vi "copyFileByFileDate.vi"() -> ()   [LabVIEW 2012]
panel:
  out "folder names":string[](array[string])
  out "filenames":string[](array[string])
  out "?":string
  out "stripped path":path
  in  "Run":bool
  out "Source":path
  out "Destination":path
  in  "path":path=path "G:/DCIM"
  in  "Target Disk":string="d:"
  in  "JPG ?":string="JPG"
  out "folder names 3":string[](array[string])
  out "filenames 3":string[](array[string])
  out "path out 3":path
  out "array":string[][](array[string])
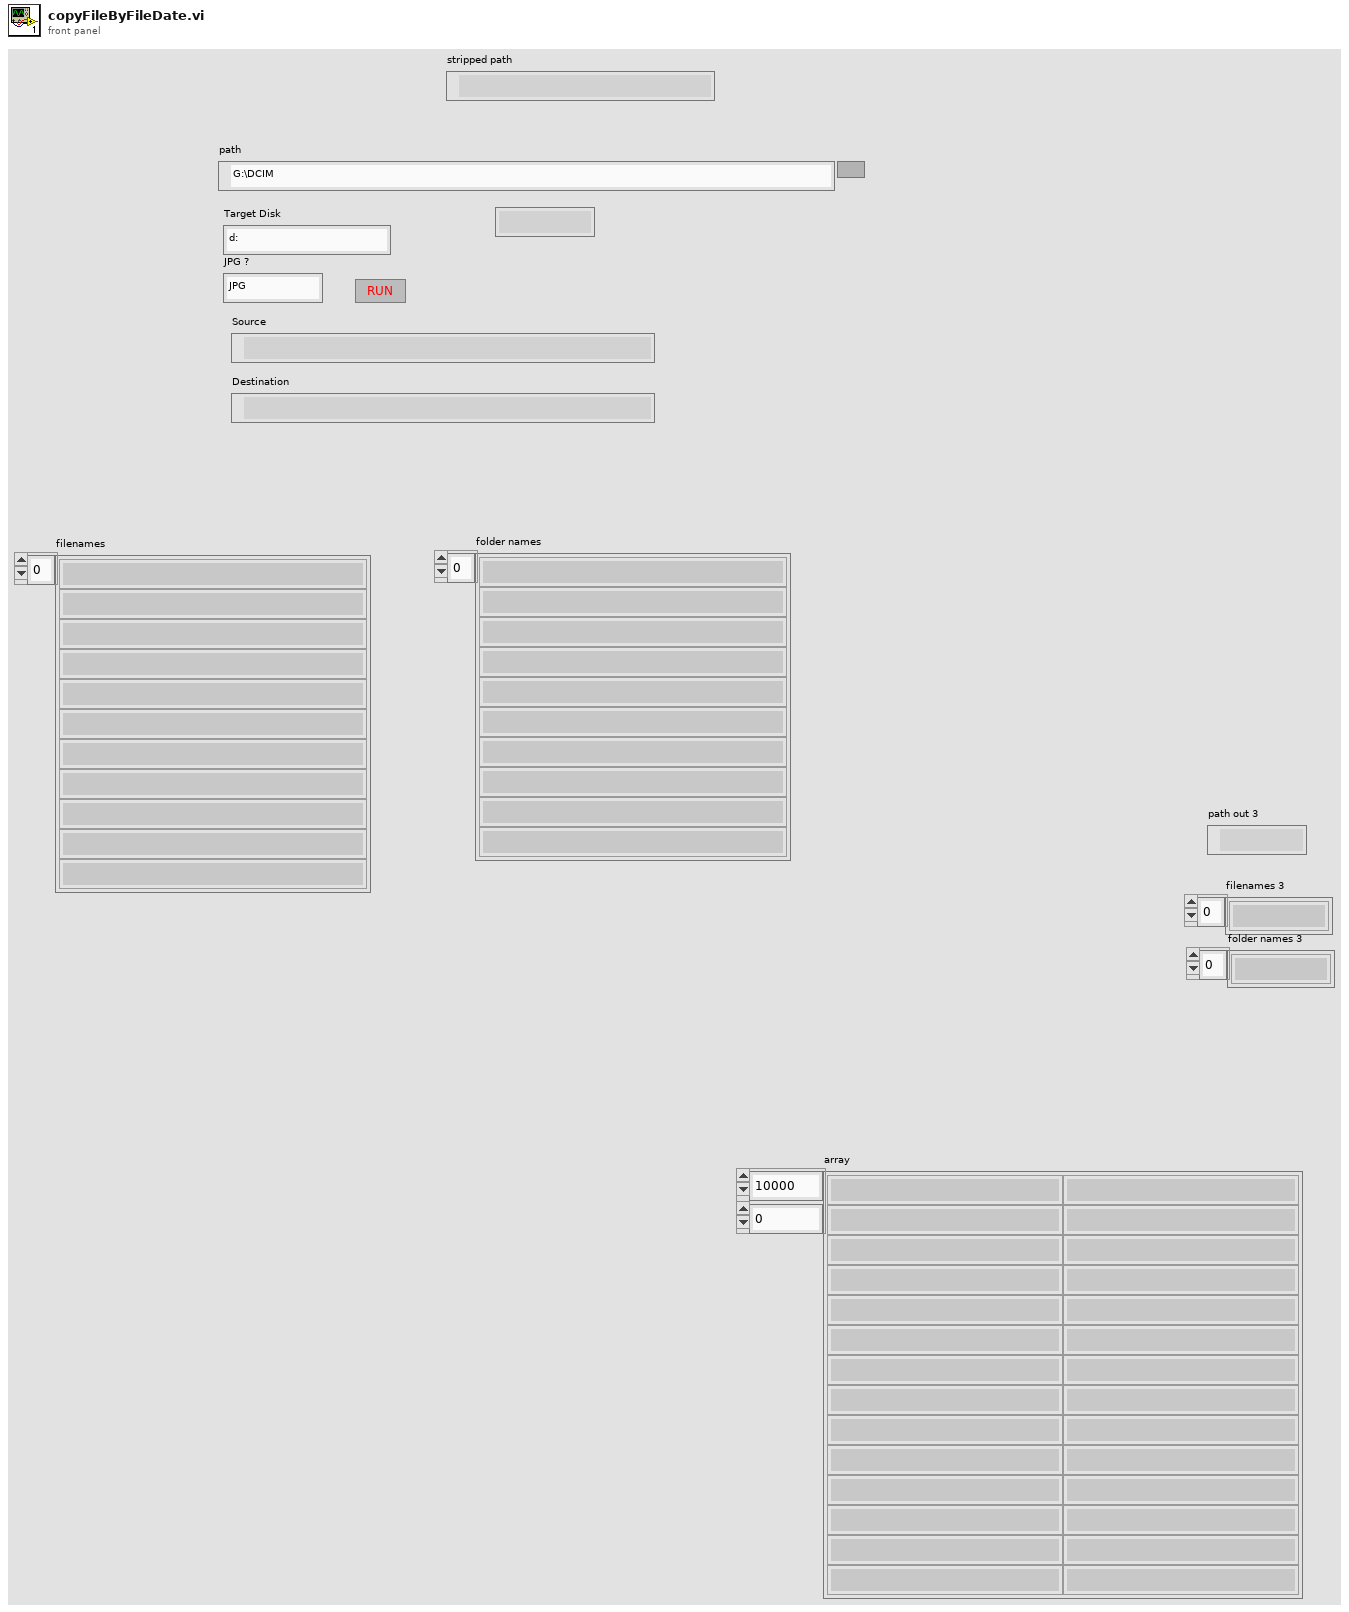
[diagram p1: front panel]
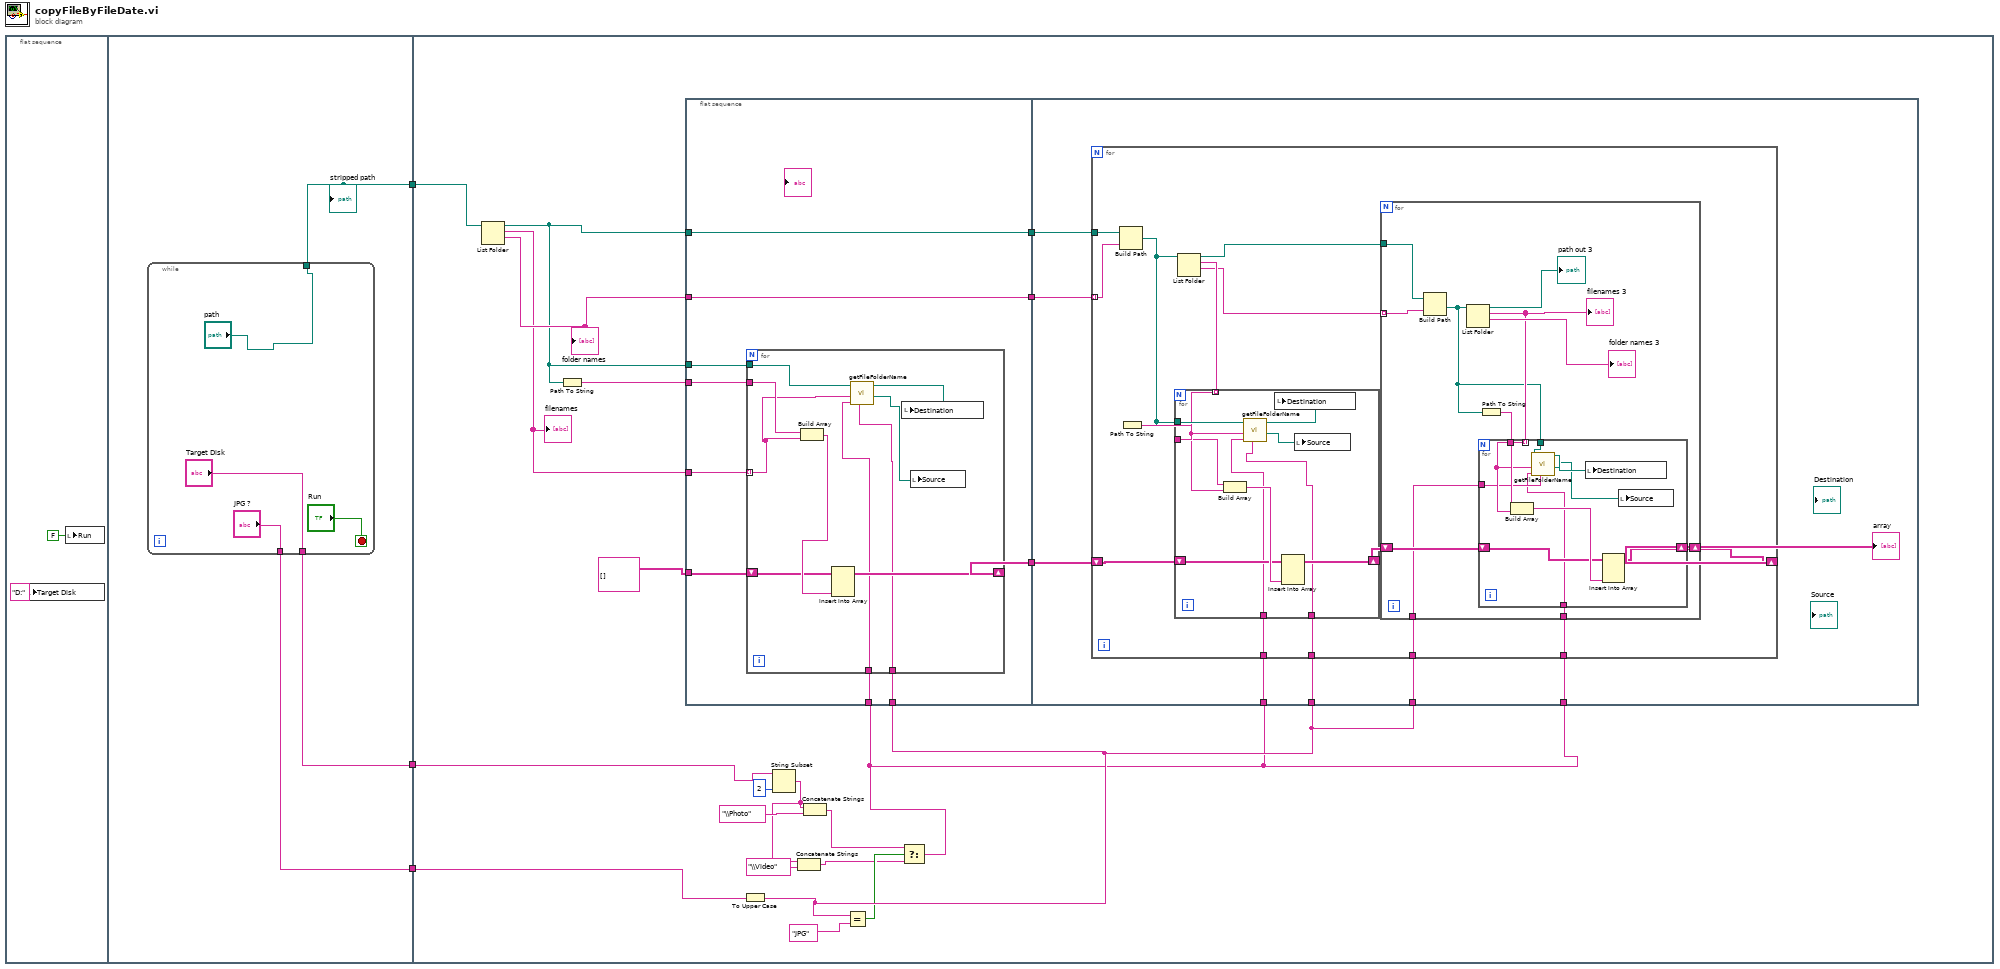
[diagram p0: block diagram]
diagram:
  n1 = flat-sequence {
    tunnel: [w8] -> w3
    tunnel: [w6] -> w2
    tunnel: [w7] -> w1
    tunnel: w3 -> [w30]
    tunnel: w2 -> [w13]
    tunnel: w1 -> [w22]
    frame #0 {
      n2 = local write "Target Disk"("D:" ("Target Disk")) -> ()
      n3 = local write "Run"(FALSE ("Run")) -> ()
    }
    frame #1 {
      n4 = while {
        tunnel: ["path"] -> w8
        tunnel: ["Target Disk"] -> w7
        tunnel: ["JPG ?"] -> w6
        stop <- "Run" stop-if-true
      }
      "stripped path" <- w8
    }
    frame #2 {
      n5 = List Folder(path=w30) -> (path out=w25:path, filenames=w26:string[], folder names=w29:string[])  [unwired: 3 in, 1 out]
      "filenames" <- w26
      "folder names" <- w29
      n6 = Path To String(path=w25) -> (string=w28:string)
      n7 = flat-sequence {
        tunnel: w25 -> [w41]
        tunnel: w29 -> [w42]
        tunnel: [w42] -> w33
        tunnel: [w41] -> w32
        tunnel: w26 -> [w40]
        tunnel: w28 -> [w39]
        tunnel: string[][] [] ("array") -> [w38]
        tunnel: [w37] -> w31
        tunnel: w25 -> [w36]
        tunnel: w23 -> [w35]
        tunnel: w17 -> [w34]
        tunnel: w33 -> [w60]
        tunnel: w32 -> [w59]
        tunnel: w31 -> [w58]
        tunnel: w23 -> [w56]
        tunnel: w23 -> [w55]
        tunnel: w17 -> [w54]
        tunnel: w17 -> [w53]
        frame #0 {
          n8 = for {
            tunnel: w40 -> [w47] mode=indexing
            tunnel: w39 -> [w52]
            shift-right: [w49] -> w37
            shift-left: w38 -> [w50]
            tunnel: w36 -> [w48]
            tunnel: w35 -> [w46]
            tunnel: w34 -> [w45]
            n9 = Build Array(w52, w47) -> (w51:string[])
            n10 = Insert Into Array(array=w50, new element=w51) -> (w49:string[][])  [unwired: 2 in]
            n11 = call "getFileFolderName.vi"("regular expression"=w46, "Directory"=w45, "name or relative path"=w47, "base path"=w48) -> ("Source"=w43:path, "Destination"=w44:path)  [unwired: 5 in, 1 out]
            n12 = local write "Destination"(w44) -> ()
            n13 = local write "Source"(w43) -> ()
          }
        }
        frame #1 {
          n14 = for {
            tunnel: w60 -> [w74] mode=indexing
            tunnel: w59 -> [w73]
            shift-right: [w68] -> w57
            shift-left: w58 -> [w66]
            tunnel: w56 -> [w64]
            tunnel: w55 -> [w63]
            tunnel: w54 -> [w62]
            tunnel: w53 -> [w61]
            n15 = Build Path(base path=w73, name or relative path=w74) -> (appended path=w65:path)
            n16 = Path To String(path=w65) -> (string=w72:string)
            n17 = List Folder(path=w65) -> (path out=w70:path, filenames=w71:string[], folder names=w69:string[])  [unwired: 3 in, 1 out]
            n18 = for {
              tunnel: w72 -> [w84]
              tunnel: w71 -> [w79] mode=indexing
              shift-right: [w82] -> w67
              shift-left: w66 -> [w81]
              tunnel: w65 -> [w80]
              tunnel: w64 -> [w78]
              tunnel: w62 -> [w77]
              n19 = Build Array(w84, w79) -> (w83:string[])
              n20 = call "getFileFolderName.vi"("regular expression"=w78, "Directory"=w77, "name or relative path"=w79, "base path"=w80) -> ("Source"=w75:path, "Destination"=w76:path)  [unwired: 5 in, 1 out]
              n21 = local write "Destination"(w76) -> ()
              n22 = Insert Into Array(array=w81, new element=w83) -> (w82:string[][])  [unwired: 2 in]
              n23 = local write "Source"(w75) -> ()
            }
            n24 = for {
              tunnel: w70 -> [w95]
              tunnel: w69 -> [w94] mode=indexing
              shift-right: [w90] -> w68
              shift-left: w67 -> [w88]
              tunnel: w63 -> [w86]
              tunnel: w61 -> [w85]
              n25 = Build Path(base path=w95, name or relative path=w94) -> (appended path=w87:path)
              n26 = List Folder(path=w87) -> (path out=→"path out 3":path, filenames=w89:string[], folder names=→"folder names 3":string[])  [unwired: 3 in, 1 out]
              "filenames 3" <- w89
              n27 = Path To String(path=w87) -> (string=w91:string)
              n28 = for {
                tunnel: w91 -> [w105]
                tunnel: w89 -> [w100] mode=indexing
                shift-right: [w103] -> w90
                shift-left: w88 -> [w102]
                tunnel: w87 -> [w101]
                tunnel: w86 -> [w99]
                tunnel: w85 -> [w98]
                n29 = Build Array(w105, w100) -> (w104:string[])
                n30 = call "getFileFolderName.vi"("regular expression"=w99, "Directory"=w98, "name or relative path"=w100, "base path"=w101) -> ("Source"=w96:path, "Destination"=w97:path)  [unwired: 5 in, 1 out]
                n31 = local write "Destination"(w97) -> ()
                n32 = Insert Into Array(array=w102, new element=w104) -> (w103:string[][])  [unwired: 2 in]
                n33 = local write "Source"(w96) -> ()
              }
            }
          }
          "array" <- w57
        }
      }
      n34 = To Upper Case(1:w13) -> (0:w23:string)
      n35 = String Subset(string=w22, length (rest)=2 ("length (rest)")) -> (substring=w15:string)  [unwired: 1 in]
      n36 = Concatenate Strings(w15, "\\Video" ("string")) -> (w16:string)
      n37 = Concatenate Strings(w15, "\\Photo" ("string")) -> (w18:string)
      n38 = Equal?(x=w23, y="JPG") -> (x = y?=w19:bool)
      n39 = Select(t=w18, s=w19, f=w16) -> (s? t:f=w17:string)
    }
  }
